vi "Execute icon editor.vi"(8 "error in (no error)":errorcluster, 10 "BW icon in":T1, 11 "Color icon in":T1) -> (0 "error out":errorcluster, 1 "Error code out":i32, 2 "BW icon out":T1, 3 "Color icon out":T1)   [LabVIEW 2021, in "IconEditorInterface.lvlib" / "IconEditorInterface.lvclass"]
uses:
  IconEditorInterface.lvclass
  <vilib>/picture/picture.llb/imagedata.ctl
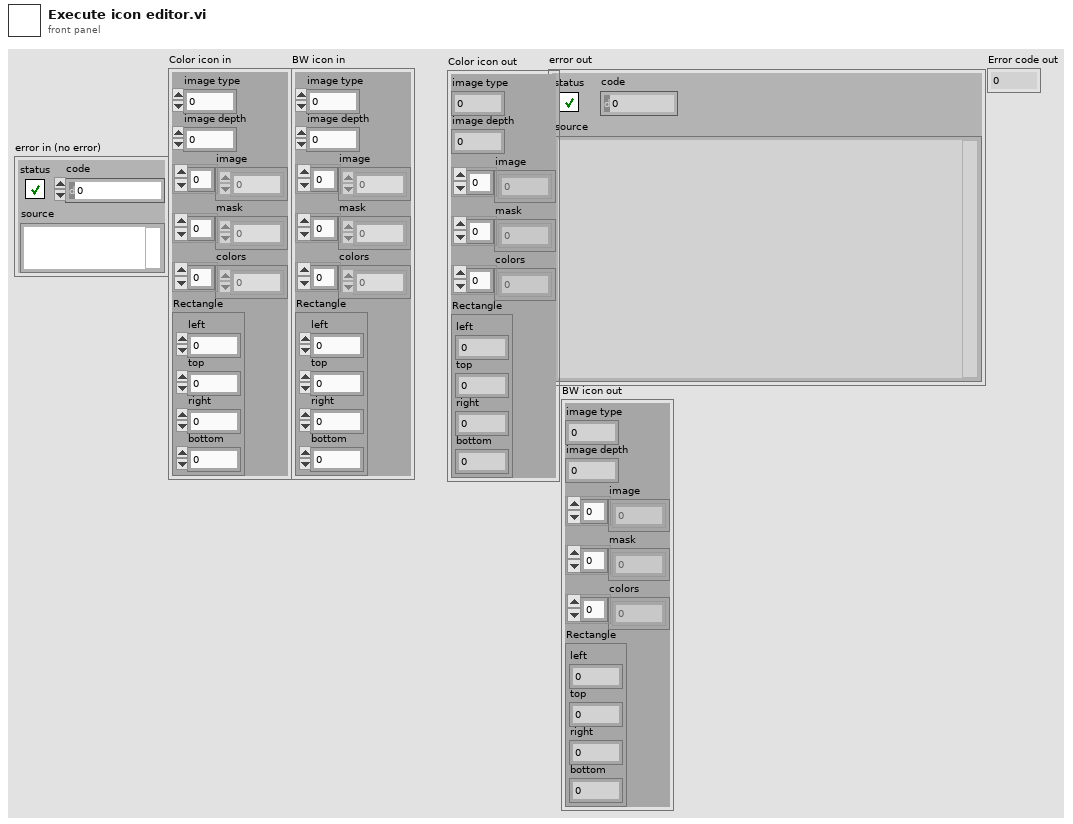
[diagram p1: front panel]
types:
  T1 = typedef "imagedata.ctl" = cluster{"image type":i32, "image depth":i32, "image":u8[], "mask":u8[], "colors":u32[], "Rectangle":cluster{"left":i16, "top":i16, "right":i16, "bottom":i16}}
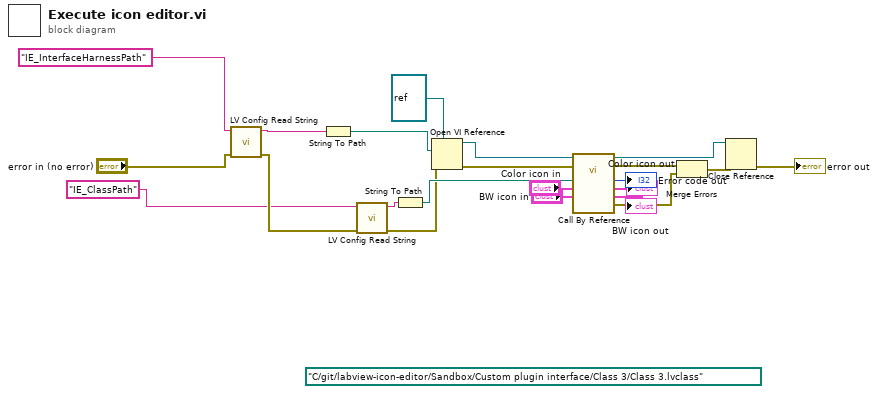
[diagram p0: block diagram]
diagram:
  (unwired) path "C:/git/labview-icon-editor/Sandbox/Custom plugin interface/Class 3/Class 3.lvclass"
  n1 = call <resource>:"LV Config Read String.vi"("error in"="error in (no error)", "key"="IE_InterfaceHarnessPath") -> ("error out"=w2:errorcluster, "value"=w15:string)  [unwired: 3 in, 1 out]
  n2 = String To Path(string=w15) -> (path=w14:path)
  n3 = call <resource>:"LV Config Read String.vi"("error in"=w2, "key"="IE_ClassPath") -> ("error out"=w5:errorcluster, "value"=w13:string)  [unwired: 3 in, 1 out]
  n4 = String To Path(string=w13) -> (path=w12:path)
  n5 = Open VI Reference(type specifier VI Refnum (for type only)=refnum<vi> refnum, vi path=w14, error in (no error)=w5) -> (vi reference=w21:refnum<vi>, error out=w22:errorcluster)  [unwired: 3 in]
  n6 = call-by-ref "?"(reference=w21, error in=w22, "BW icon in"="BW icon in", "Color icon in"="Color icon in", "Class"=w12) -> (reference out=w18:refnum<vi>, error out=w17:errorcluster, 0:"error out"=w11:errorcluster, "BW icon out"=→"BW icon out":T1, "Color icon out"=→"Color icon out":T1, "Error code out"=→"Error code out":i32)  [unwired: 5 in]
  n7 = Merge Errors(w17, w11) -> (w16:errorcluster)
  n8 = Close Reference(reference=w18, error in (no error)=w16) -> (error out=→"error out":errorcluster)
